vi "Launch DQMH Tools by menu.vi"(8 "error in":errorcluster, 9 "DQMH Tools":T2, 10 "Current Selection In":T1, 11 "Project In":refnum<class "Project.lvclass">) -> (0 "error out":errorcluster, 3 "Project Out":refnum<class "Project.lvclass">)   [LabVIEW 2020, in "Panther Dashboard.lvlib"]
doc: "Launch a DQMH scripting tool by typing one of the following strings in Quick Drop before pressing the Ctrl-Key shortcut for this plugin:\n\nCreate New DQMH Event - ae, new event, add event, create event, \"\" (empty string)\nRename DQMH Event - re, rename event\nRemove DQMH Event - rme, remove\nConvert DQMH Event - ce, convert\nAdd New DQMH Module - am, new mod, add mod, create mod\nRename DQMH Module - rm, rename module\nValidate DQMH Module - vm, validate\nCreate DQMH Module Template - ct, template\nCreate RT Tester - crt, rt\nNew DQMH Unit Test - cut, unit\n\nDefault Shortcut - [E]"
uses:
  Panther Dashboard.lvlib
  DQMH Tools Menu--enum.ctl
  Class/Project/Project.lvclass
  Class/Library/Library.lvclass
  C:/GitClones/PantherDashboard/src/LabVIEW/Panther Dashboard/Class/LabVIEWItem/LabVIEWItem.lvclass
  Class/VI/VI.lvclass
  Class/LabVIEWItem/LabVIEWItem.lvclass/LabVIEWItem.ctl
  Class/LabVIEWItem/Read Item Path.vi
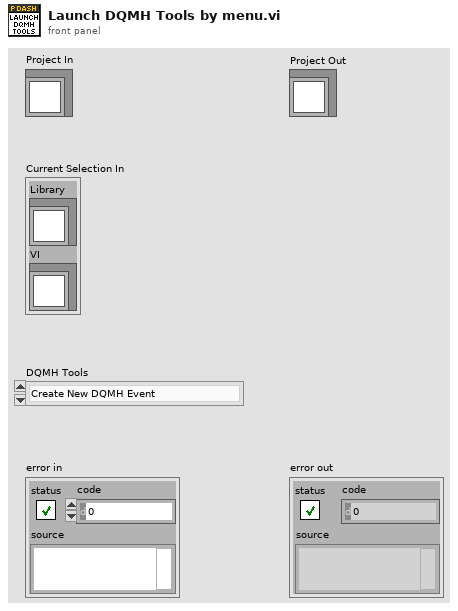
[diagram p1: front panel]
types:
  T1 = cluster{"Library":refnum<class "Library.lvclass">, "VI":refnum<class "VI.lvclass">}
  T2 = typedef "Panther Dashboard.lvlib/DQMH Tools Menu--enum.ctl" = enum16{"Create New DQMH Event", "Remove DQMH Event", "Convert DQMH Event", "Rename DQMH Event", "Add New DQMH Module", "Create RT Tester", "Rename DQMH Module", "Validate DQMH Module", "Create DQMH Module Template", "New DQMH  Unit Test", "Add Helper Loop to DQMH Module", "Duplicate Event", "HSE-ify DQMH Module", "Duplicate Module"}
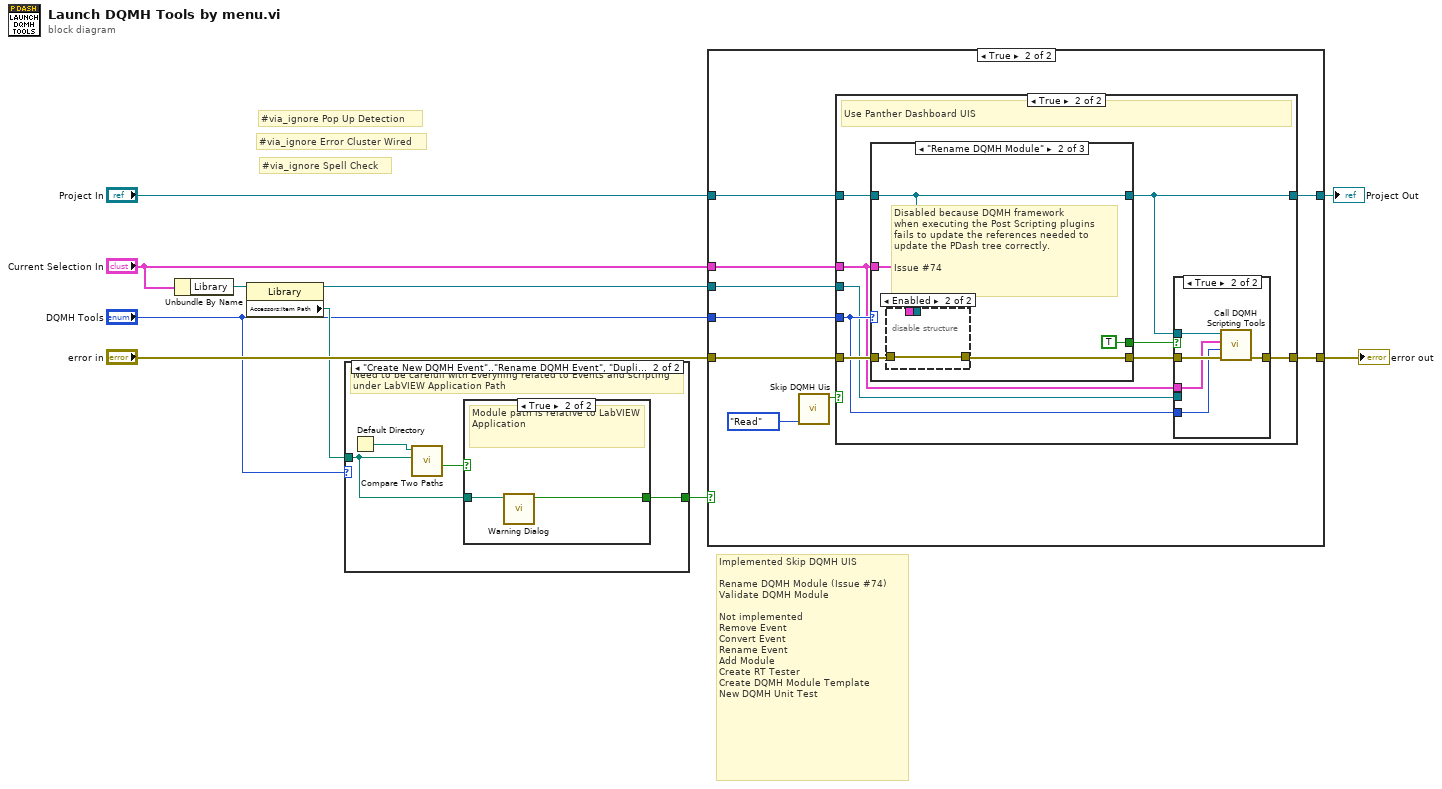
[diagram p0: block diagram]
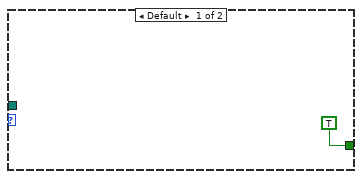
[diagram p2: hidden frame]
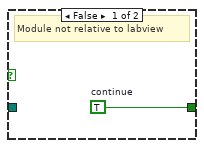
[diagram p3: hidden frame]
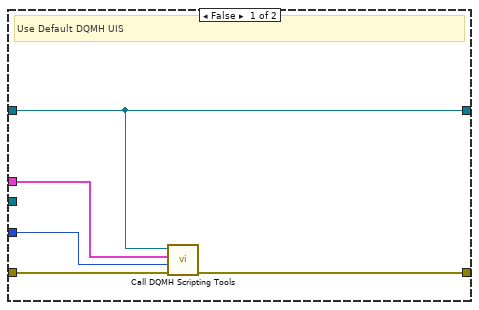
[diagram p5: hidden frame]
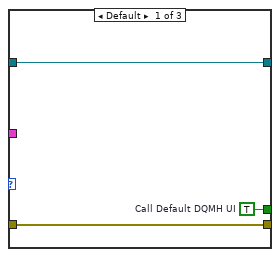
[diagram p7: hidden frame]
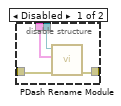
[diagram p8: hidden frame]
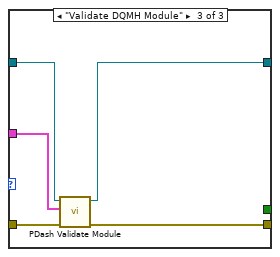
[diagram p9: hidden frame]
diagram:
  # "Implemented Skip DQMH UIS\n\nRename DQMH Module (Issue #74)\nValidate DQMH Module\n\nNot implemented \nRemove Event\nConvert Event\nRename Event\nAdd Module\nCreate RT Tester\nCreate DQMH Module Template\nNew DQMH Unit Test"
  # "#via_ignore Error Cluster Wired"
  # "#via_ignore Pop Up Detection"
  # "#via_ignore Spell Check"
  n1 = Unbundle By Name("Current Selection In") -> ("Library"=w5:refnum<class "Library.lvclass">)
  n2 = property class="Library"(reference=w5) -> (reference out=w3:refnum<class "Library.lvclass">, "Accessors:Item Path"=w6:path)  [unwired: 1 in, 1 out]
  n3 = case shown="\"Create New DQMH Event\"..\"Rename DQMH Event\", \"Duplicate Event\"" "DQMH Tools" {
    tunnel: [TRUE ("Continue?") w15] -> w8
    tunnel: w6 -> [_ w13]
    frame Default {
    }
    frame "Create New DQMH Event".."Rename DQMH Event", "Duplicate Event" {
      # "Need to be carefull with Everyhing related to Events and scripting under LabVIEW Application Path"
      n4 = Default Directory() -> (w12:path)
      n5 = call <vilib>:"Compare Two Paths.vi"("Path 2"=w13, "Path 1"=w12) -> ("Path 2 Relative to Path 1?"=w14:bool)  [unwired: 6 in, 3 out]
      n6 = case shown="True" w14 {
        tunnel: [w16 w18] -> w15
        tunnel: w13 -> [_ w17]
        frame False {
          w16 = TRUE  # continue
          # "Module not relative to labview"
        }
        frame True {
          # "Module path is relative to LabVIEW Application"
          n7 = call "Warning Dialog.vi"("Path"=w17) -> ("Continue?"=w18:bool)  [unwired: 10 in]
        }
      }
    }
  }
  n8 = case shown="True" w8 {
    tunnel: "DQMH Tools" -> [_ w27]
    tunnel: "Project In" -> [w19 w25]
    tunnel: "Current Selection In" -> [_ w24]
    tunnel: "error in" -> [w20 w29]
    tunnel: [w20 w28] -> w10
    tunnel: w3 -> [_ w22]
    tunnel: [w19 w21] -> w1
    frame False {
      # "The Selection Path is relative to LabVIEW Application and User Canceled action"
    }
    frame True {
      n9 = call "Skip DQMH Uis.vi"("Action"=enum16{"Read", "Write", "Delete"}."Read") -> ("Skip DQMH UIs"=w26:bool)  [unwired: 10 in]
      n10 = case shown="True" w26 {
        tunnel: w27 -> [w32 w38]
        tunnel: w25 -> [w30 w40]
        tunnel: w24 -> [w31 w36]
        tunnel: w29 -> [w33 w43]
        tunnel: [w34 w41] -> w28
        tunnel: w22 -> [_ w37]
        tunnel: [w30 w35] -> w21
        frame False {
          # "Use Default DQMH UIS"
          n11 = call "Call DQMH Scripting Tools.vi"("error in"=w33, "DQMH Tools"=w32, "Current Selection In"=w31, "Project in"=w30) -> ("error out"=w34:errorcluster)  [unwired: 7 in]
        }
        frame True {
          # "Use Panther Dashboard UIS"
          n12 = case shown="\"Rename DQMH Module\"" w38 {
            tunnel: w40 -> [w51 w55 w64]
            tunnel: w36 -> [_ w54 w65]
            tunnel: w43 -> [w52 w57 w67]
            tunnel: [w52 w56 w66] -> w42
            tunnel: [w51 w55 w63] -> w35
            tunnel: [w50 TRUE ("Call Default DQMH UI") _] -> w39
            frame Default {
              w50 = TRUE  # Call Default DQMH UI
            }
            frame "Rename DQMH Module" {
              # "Disabled because DQMH framework\nwhen executing the Post Scripting plugins\nfails to update the references needed to\nupdate the PDash tree correctly.\n\nIssue #74"
              n13 = disable-structure shown="Enabled" {
                disable-tunnel: w57 -> [w61 w62]
                disable-tunnel: [w60 w62] -> w56
                disable-tunnel: w55 -> [w59 _]
                disable-tunnel: w54 -> [w58 _]
                frame Disabled {
                  n14 = call "PDash Rename Module.vi"("error in"=w61, "Current Selection"=w58, "Project"=w59) -> ("error out"=w60:errorcluster)  [unwired: 8 in]
                }
                frame Enabled {
                }
              }
            }
            frame "Validate DQMH Module" {
              n15 = call "PDash Validate Module.vi"("error in"=w67, "Current Selection"=w65, "Project"=w64) -> ("error out"=w66:errorcluster, "Project Out"=w63:refnum<class "Project.lvclass">)  [unwired: 7 in]
            }
          }
          n16 = case shown="True" w39 {
            tunnel: w35 -> [_ w47]
            tunnel: w38 -> [_ w46]
            tunnel: w42 -> [w44 w49]
            tunnel: [w44 w48] -> w41
            tunnel: w37 -> [_ _]
            tunnel: w36 -> [_ w45]
            frame False {
            }
            frame True {
              n17 = call "Call DQMH Scripting Tools.vi"("error in"=w49, "DQMH Tools"=w46, "Current Selection In"=w45, "Project in"=w47) -> ("error out"=w48:errorcluster)  [unwired: 7 in]
            }
          }
        }
      }
    }
  }
  "error out" <- w10
  "Project Out" <- w1
